vi "Read Waveform (Single).vi"(8 "error in (no error)":errorcluster, 9 "Maximum Time (10000 ms)":u32=10000, 10 "Channel (1: Channel 1)":u16(ring)=1 items=["Channel 1"=1, "Channel 2"=2, "Channel 3"=3, "Channel 4"=4], 11 "VISA resource name":refnum<visa-resource-name>) -> (0 "error out":errorcluster, 2 "Waveform Data":waveform(dbl)(graph), 3 "VISA resource name out":refnum<visa-resource-name>)   [LabVIEW 2011, in "Agilent DSO1000 Series.lvlib"]
doc: "Initiates an acquisition on all channels that you enabled with the Configure Channel VI. The VI waits for the acquisition to complete and returns the waveform for the <B>Source Channel</B> you specified. If the oscilloscope did not complete the acquisition within the time period you specify with the <B>Timeout</B> control, the VI returns a timeout error. A common cause for a timeout error is the acquisition was not triggered. For example, the trigger level is out of range of the waveform.\n\nCall the Fetch Waveform VI to obtain the waveforms for each of the remaining enabled <B>Source Channels</B> without initiating another acquisition.\n\n<B>Note:</B> If your instrument does not support auto compensation for probe attenuation, you may need to adjust the scaling of the Waveform Data accordingly. This is handled automatically in the <B>Configure Channel</B> VI or can be done manually by multiplying the <B>Waveform Data</B> by the probe attenuation."
uses:
  <instrlib>/Agilent DSO1000 Series/Agilent DSO1000 Series.lvlib
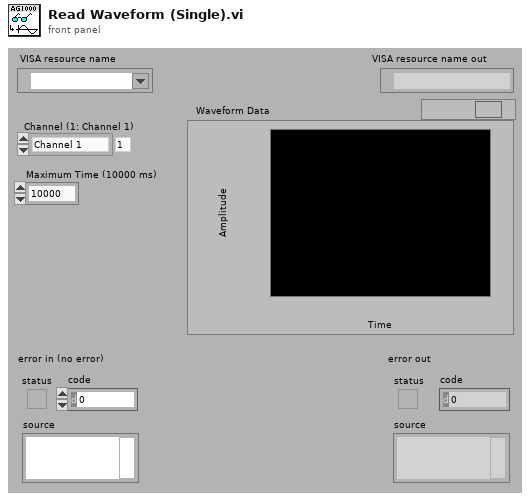
[diagram p1: front panel]
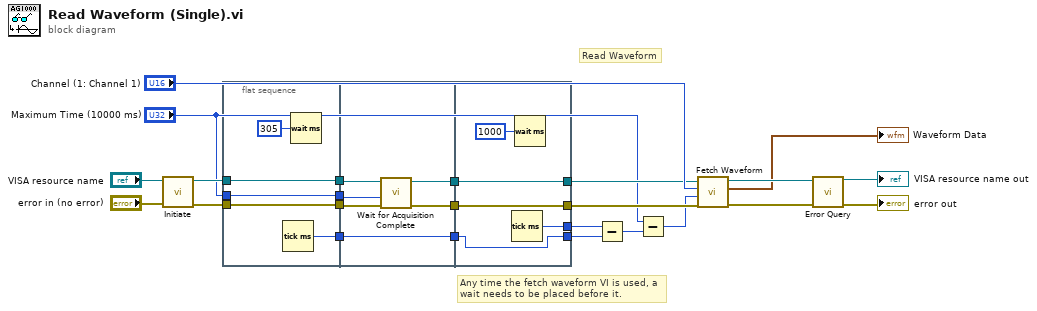
[diagram p0: block diagram]
diagram:
  # "Any time the fetch waveform VI is used, a wait needs to be placed before it."
  # "Read Waveform"
  n1 = call <instrlib>:"Initiate.vi"("error in (no error)"="error in (no error)", "VISA resource name"="VISA resource name") -> ("error out"=w14:errorcluster, "VISA resource name out"=w16:refnum<visa-resource-name>)  [unwired: 8 in]
  n2 = flat-sequence {
    tunnel: w16 -> [w28]
    tunnel: [w28] -> w7
    tunnel: w14 -> [w27]
    tunnel: [w27] -> w6
    tunnel: "Maximum Time (10000 ms)" -> [w26]
    tunnel: [w26] -> w5
    tunnel: [w29] -> w4
    tunnel: w7 -> [w35]
    tunnel: [w34] -> w3
    tunnel: w6 -> [w33]
    tunnel: [w32] -> w2
    tunnel: w5 -> [w31]
    tunnel: w4 -> [w30]
    tunnel: [w30] -> w1
    tunnel: [w39] -> w15
    tunnel: w3 -> [w39]
    tunnel: [w38] -> w13
    tunnel: w2 -> [w38]
    tunnel: [w37] -> w9
    tunnel: w1 -> [w37]
    tunnel: [w40] -> w8
    frame #0 {
      n3 = Tick Count (ms)() -> (millisecond timer value=w29:u32)
      n4 = Wait (ms)(milliseconds to wait=u32 305) -> ()  [unwired: 1 out]
    }
    frame #1 {
      n5 = call <instrlib>:"Wait for Acquisition Complete.vi"("error in (no error)"=w33, "Maximum Time (10000 ms)"=w31, "VISA resource name"=w35) -> ("error out"=w32:errorcluster, "VISA resource name out"=w34:refnum<visa-resource-name>)  [unwired: 7 in]
    }
    frame #2 {
      n6 = Tick Count (ms)() -> (millisecond timer value=w40:u32)
      n7 = Wait (ms)(milliseconds to wait=u32 1000) -> ()  [unwired: 1 out]
    }
  }
  n8 = Subtract(x=w8, y=w9) -> (x-y=w12:u32)
  n9 = Subtract(x="Maximum Time (10000 ms)", y=w12) -> (x-y=w10:u32)
  n10 = call <instrlib>:"Fetch Waveform.vi"("error in (no error)"=w13, "Maximum Time (10000 ms)"=w10, "Channel (1: Channel 1)"="Channel (1: Channel 1)", "VISA resource name"=w15) -> ("error out"=w18:errorcluster, "Waveform Data"=→"Waveform Data":waveform(dbl), "VISA resource name out"=w19:refnum<visa-resource-name>)  [unwired: 5 in]
  n11 = call <instrlib>:"Error Query.vi"("error in (no error)"=w18, "VISA resource name"=w19) -> ("error out"=→"error out":errorcluster, "VISA resource name out"=→"VISA resource name out":refnum<visa-resource-name>)  [unwired: 6 in, 2 out]
